vi "Zero Crossing.vi"(0 "waveforms in":waveform(dbl)[](array[waveform]), 1 "reset? (F)":bool, 9 "system info in":refnum<class "EP System Info.lvclass">, 11 "error in (no error)":errorcluster) -> (4 "waveforms out":waveform(dbl)[](array[waveform]), 6 "zero crossings":cluster{"zero crossing":dbl[]}[](array[cluster]), 8 "samples since the last cross":cluster{"samples since the last cross":dbl[]}[](array[cluster]), 10 "system info out":refnum<class "EP System Info.lvclass">, 15 "error out":errorcluster)   [LabVIEW 2014, in "NI_EP_Power Quality.lvlib"]
doc: "Calculates the zero crossing indexes for voltage waveforms, current waveforms, or waveforms that contain both voltage and current. Zero crossing is the instantaneous point at which the voltage or current turns from positive to negative or from negative to positive.\n\nThis VI supports measuring single-line and multiple-line systems."
uses:
  <vilib>/addons/Electrical Power/PQ/NI_EP_Power Quality.lvlib
  <vilib>/addons/Electrical Power/PQ/Common/Classes/System Info/EP System Info.lvclass
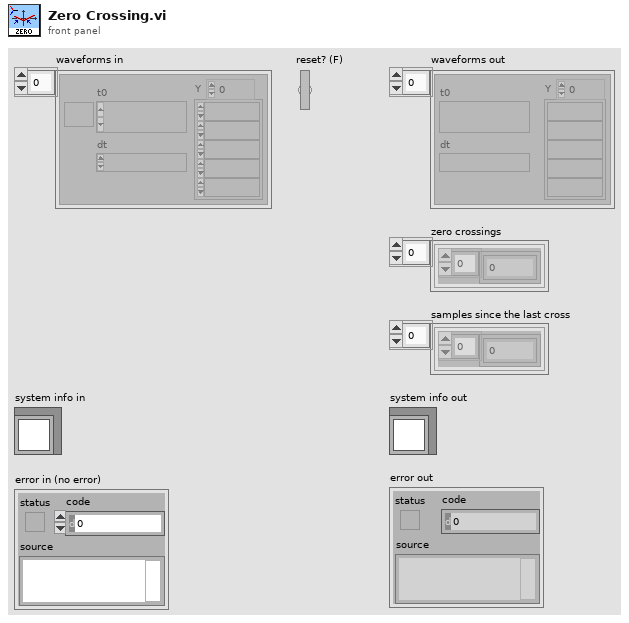
[diagram p1: front panel]
types:
  T1 = cluster{"filter structure":enum32{"IIR 2nd Order", "IIR 4th Order"}, "Reverse Coefficients":dbl[], "Forward Coefficients":dbl[]}
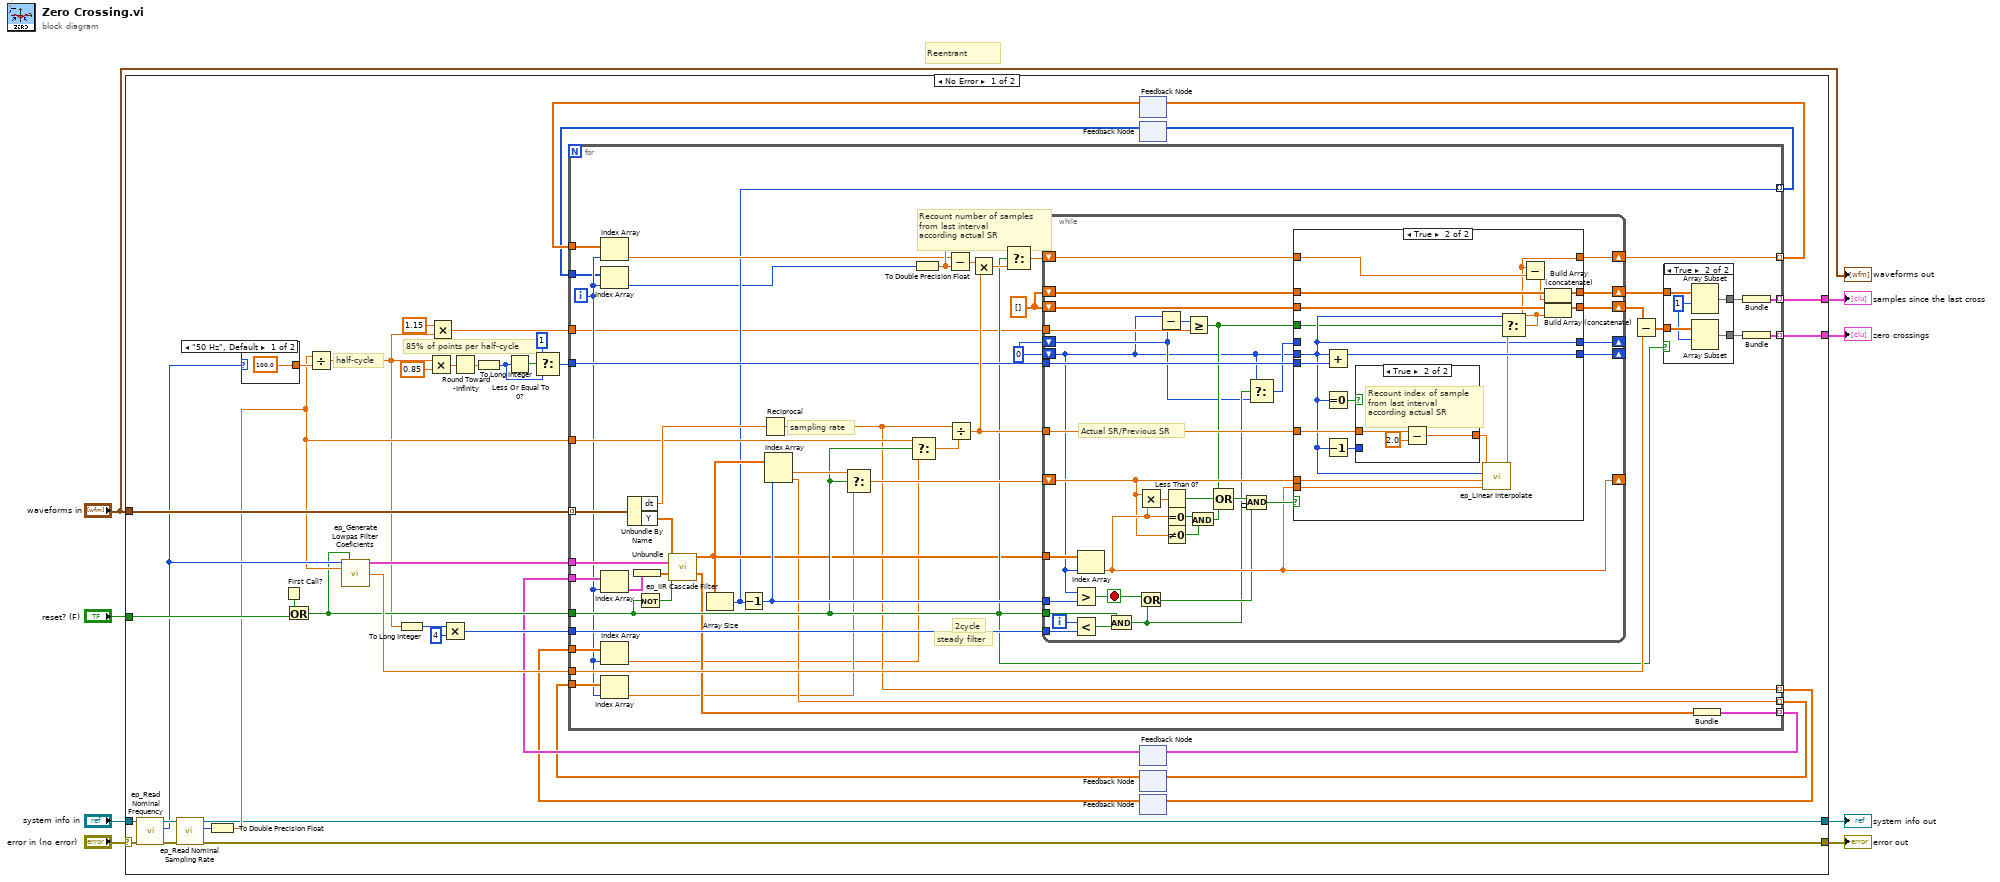
[diagram p0: block diagram]
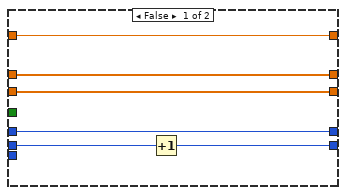
[diagram p3: hidden frame]
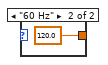
[diagram p5: hidden frame]
diagram:
  # "Reentrant"
  n1 = case shown="No Error" "error in (no error)" {
    selector: "error in (no error)" -> [w28 w170]
    tunnel: "waveforms in" -> [w49 _]
    tunnel: [w44 _] -> w8
    tunnel: [w43 _] -> w7
    tunnel: [w27 w170] -> w5
    tunnel: "reset? (F)" -> [w36 _]
    tunnel: "system info in" -> [w26 w169]
    tunnel: [w23 w169] -> w2
    frame No Error {
      # "85% of points per half-cycle"
      # "half-cycle"
      n2 = call <vilib>:"ep_Read Nominal Frequency.vi"("error in (no error)"=w28, "system info in"=w26) -> ("error out"=w30:errorcluster, "nominal frequency"=w25:enum16{"50 Hz", "60 Hz"}, "system info out"=w29:refnum<class "EP System Info.lvclass">)  [unwired: 6 in, 1 out]
      n3 = call <vilib>:"ep_Read Nominal Sampling Rate.vi"("error in (no error)"=w30, "system info in"=w29) -> ("error out"=w27:errorcluster, "nominal sampling rate (Hz)"=w31:u16, "system info out"=w23:refnum<class "EP System Info.lvclass">)  [unwired: 7 in]
      n4 = To Double Precision Float(number=w31) -> (double precision float=w24:dbl)
      n5 = case shown="\"50 Hz\", Default" w25 {
        tunnel: [100.0 ("y") 120.0 ("y")] -> w48
        frame "50 Hz", Default {
        }
        frame "60 Hz" {
        }
      }
      n6 = First Call?() -> (First Call?: T/F=w35:bool)
      n7 = Or(x=w35, y=w36) -> (x .or. y?=w22:bool)
      n8 = Divide(x=w24, y=w48) -> (x/y=w10:dbl)
      n9 = call <vilib>:"ep_Generate Lowpas Filter Coeficients.vi"("nominal frequency"=w25, "restart (F)"=w22, "nominal sampling rate (Hz)"=w24) -> ("IIR filter cluster"=w42:T1, "filter delay (samples)"=w41:dbl)  [unwired: 11 in]
      n10 = To Long Integer(number=w10) -> (32bit integer=w45:i32)
      n11 = Multiply(x=w10, y=0.85) -> (x*y=w34:dbl)
      n12 = Multiply(x=1.15 ("y"), y=w10) -> (x*y=w9:dbl)
      n13 = Multiply(x=w45, y=4) -> (x*y=w47:i32)
      n14 = Round Toward -Infinity(1:w34) -> (0:w32:dbl)
      n15 = To Long Integer(number=w32) -> (32bit integer=w37:i32)
      n16 = Less Or Equal To 0?(x=w37) -> (x <= 0?=w40:bool)
      n17 = Select(t=1, s=w40, f=w37) -> (s? t:f=w38:i32)
      n18 = feedback #1() -> (w20:dbl[])  [unwired: 1 in]
      n19 = feedback #2() -> (w12:i32[])  [unwired: 1 in]
      n20 = feedback #3() -> (w18:cluster{"shift register out":dbl[]}[])  [unwired: 1 in]
      n21 = feedback #4() -> (w16:dbl[])  [unwired: 1 in]
      n22 = feedback #5() -> (w14:dbl[])  [unwired: 1 in]
      n23 = for {
        tunnel: w49 -> [w96] mode=indexing
        tunnel: w47 -> [w93]
        tunnel: [w75] -> w44 mode=indexing
        tunnel: [w74] -> w43 mode=indexing
        tunnel: w42 -> [w71]
        tunnel: w41 -> [w90]
        tunnel: w38 -> [w89]
        tunnel: w24 -> [w77]
        tunnel: w22 -> [w76]
        tunnel: [w73] -> w21 mode=indexing
        tunnel: w20 -> [w68]
        tunnel: w18 -> [w64]
        tunnel: [w65] -> w19 mode=indexing
        tunnel: [w61] -> w17 mode=indexing
        tunnel: w16 -> [w60]
        tunnel: [w58] -> w15 mode=indexing
        tunnel: w14 -> [w57]
        tunnel: [w55] -> w13 mode=indexing
        tunnel: w12 -> [w53]
        tunnel: w9 -> [w50]
        i -> [w54]
        w85 = dbl[] []
        w51 = 0
        # "Recount number of samples\nfrom last interval\naccording actual SR"
        # "steady filter"
        # "2cycle"
        # "sampling rate"
        n24 = Index Array(array=w68, index=w54) -> (element=w67:dbl)
        n25 = Index Array(array=w53, index=w54) -> (element=w52:i32)
        n26 = Index Array(array=w64, index=w54) -> (element=w63:cluster{"shift register out":dbl[]})
        n27 = Index Array(array=w57, index=w54) -> (element=w56:dbl)
        n28 = Index Array(array=w60, index=w54) -> (element=w59:dbl)
        n29 = Unbundle By Name(w96) -> ("dt"=w95:dbl, "Y"=w69:dbl[])
        n30 = Unbundle(w63) -> ("shift register out"=w62:dbl[])
        n31 = Not(x=w76) -> (.not. x?=w70:bool)
        n32 = call <vilib>:"ep_IIR Cascade Filter.vi"("X"=w69, "IIR Filter Cluster"=w71, "shift register in"=w62, "init/cont (init:F)"=w70) -> ("Filtered X"=w72:dbl[], "shift register out"=w66:dbl[])  [unwired: 9 in, 1 out]
        n33 = Array Size(array=w72) -> (size(s)=w55:i32)
        n34 = Decrement(x=w55) -> (x-1=w97:i32)
        n35 = Reciprocal(x=w95) -> (1/x=w58:dbl)
        n36 = Index Array(array=w72, index #2=w97) -> (element #1=w87:dbl, element #2=w61:dbl)  [unwired: 1 in]
        n37 = Select(t=w87, s=w76, f=w59) -> (s? t:f=w88:dbl)
        n38 = Select(t=w77, s=w76, f=w56) -> (s? t:f=w86:dbl)
        n39 = To Double Precision Float(number=w52) -> (double precision float=w78:dbl)
        n40 = Subtract(x=w67, y=w78) -> (x-y=w84:dbl)
        n41 = Divide(x=w58, y=w86) -> (x/y=w94:dbl)
        n42 = Multiply(x=w84, y=w94) -> (x*y=w80:dbl)
        n43 = Select(t=w78, s=w76, f=w80) -> (s? t:f=w79:dbl)
        n44 = while {
          shift-right: [w137] -> w81
          shift-left: w85 -> [w135]
          shift-right: [w131] -> _
          shift-left: w88 -> [w113]
          tunnel: w72 -> [w138]
          tunnel: w97 -> [w133]
          shift-right: [w136] -> _
          shift-left: w51 -> [w105]
          tunnel: w89 -> [w134]
          tunnel: w94 -> [w130]
          shift-right: [w129] -> w73
          shift-left: w79 -> [w128]
          shift-right: [w126] -> w83
          shift-left: w85 -> [w127]
          tunnel: w76 -> [w123]
          tunnel: w93 -> [w121]
          shift-right: [w110] -> _
          shift-left: w51 -> [w106]
          tunnel: w50 -> [w111]
          i -> [w122]
          stop <- w125 stop-if-true
          # "Actual SR/Previous SR"
          n45 = Greater?(x=w105, y=w133) -> (0:w125:bool)
          n46 = Less?(x=w122, y=w121) -> (x < y?=w124:bool)
          n47 = Index Array(array=w138, index=w105) -> (element=w131:dbl)
          n48 = And(x=w123, y=w124) -> (x .and. y?=w108:bool)
          n49 = Multiply(x=w113, y=w131) -> (x*y=w120:dbl)
          n50 = Or(x=w125, y=w108) -> (x .or. y?=w114:bool)
          n51 = Subtract(x=w105, y=w106) -> (x-y=w112:i32)
          n52 = Less Than 0?(x=w120) -> (x < 0?=w117:bool)
          n53 = Equal To 0?(x=w131) -> (x = 0?=w119:bool)
          n54 = Not Equal To 0?(x=w113) -> (x != 0?=w118:bool)
          n55 = Greater Or Equal?(x=w112, y=w111) -> (x >= y?=w109:bool)
          n56 = And(x=w119, y=w118) -> (x .and. y?=w116:bool)
          n57 = Compound Arithmetic op=OR(w109, w117, w116) -> (w115:bool)
          n58 = Compound Arithmetic op=AND(w115, invert w114) -> (w132:bool)
          n59 = Select(t=w105, s=w108, f=w106) -> (s? t:f=w107:i32)
          n60 = case shown="True" w132 {
            tunnel: w135 -> [w144 w162]
            tunnel: [w144 w161] -> w137
            tunnel: w105 -> [w143 w146]
            tunnel: [w142 w155] -> w136
            tunnel: w134 -> [_ w160]
            tunnel: w113 -> [_ w159]
            tunnel: w131 -> [_ w158]
            tunnel: w130 -> [_ w154]
            tunnel: [w141 w147] -> w129
            tunnel: w128 -> [w141 w153]
            tunnel: w127 -> [w140 w152]
            tunnel: [w140 w150] -> w126
            tunnel: w109 -> [_ w145]
            tunnel: w107 -> [w139 _]
            tunnel: [w139 w146] -> w110
            frame False {
              n61 = Increment(x=w143) -> (x+1=w142:i32)
            }
            frame True {
              n62 = Add(x=w146, y=w160) -> (x+y=w155:i32)
              n63 = Equal To 0?(x=w146) -> (x = 0?=w157:bool)
              n64 = Decrement(x=w146) -> (x-1=w156:i32)
              n65 = case shown="True" w157 {
                tunnel: w156 -> [w163 _]
                tunnel: [w163 w164] -> w149
                tunnel: w154 -> [_ w166]
                frame False {
                }
                frame True {
                  # "Recount index of sample\nfrom last interval\naccording actual SR"
                  n66 = Subtract(x=w166, y=2.0) -> (x-y=w164:dbl)
                }
              }
              n67 = call <vilib>:"ep_Linear Interpolate.vi"("y2"=w158, "y1"=w159, "x2"=w146, "x1"=w149) -> ("y"=w148:dbl)  [unwired: 7 in]
              n68 = Select(t=w146, s=w145, f=w148) -> (s? t:f=w147:dbl)
              n69 = Subtract(x=w147, y=w153) -> (x-y=w151:dbl)
              n70 = Build Array (concatenate)(w152, w151) -> (w150:dbl[])
              n71 = Build Array (concatenate)(w162, w147) -> (w161:dbl[])
            }
          }
        }
        n72 = Subtract(x=w81, y=w90) -> (x-y=w82:dbl[])
        n73 = case shown="True" w76 {
          tunnel: w83 -> [w98 w104]
          tunnel: [w98 w103] -> w92
          tunnel: w82 -> [w99 w102]
          tunnel: [w99 w101] -> w91
          frame False {
          }
          frame True {
            w100 = 1 ("index")
            n74 = Array Subset(array=w104, index=w100) -> (w103:dbl[])  [unwired: 1 in]
            n75 = Array Subset(array=w102, index=w100) -> (w101:dbl[])  [unwired: 1 in]
          }
        }
        n76 = Bundle("shift register out"=w66) -> (w65:cluster{"shift register out":dbl[]})  [unwired: 1 in]
        n77 = Bundle(w92) -> (w75:cluster{dbl[]})  [unwired: 1 in]
        n78 = Bundle(w91) -> (w74:cluster{dbl[]})  [unwired: 1 in]
      }
      n79 = feedback-in #1(w21) -> ()
      n80 = feedback-in #2(w13) -> ()
      n81 = feedback-in #3(w19) -> ()
      n82 = feedback-in #4(w17) -> ()
      n83 = feedback-in #5(w15) -> ()
    }
    frame Error {
    }
  }
  "error out" <- w5
  "zero crossings" <- w7
  "samples since the last cross" <- w8
  "system info out" <- w2
  "waveforms out" <- "waveforms in"
